vi "UI.vi"() -> ()   [LabVIEW 2017, in "TestLibrary.lvlib" / "GSharpCls.lvclass"]
uses:
  GSharpCls.lvclass
  Enum.ctl
panel:
  out "error out":errorcluster
  in  "Enum":T1
  out "Numeric out":dbl
  out "String":string
  in  "Numeric":dbl
  in  "stop":bool
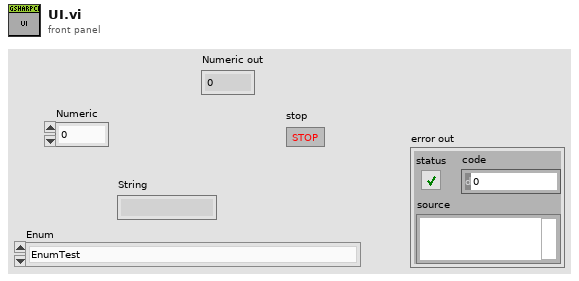
[diagram p1: front panel]
types:
  T1 = typedef "TestLibrary.lvlib/GSharpCls.lvclass/Enum.ctl" = enum16{"EnumTest", "EnumTest2"}
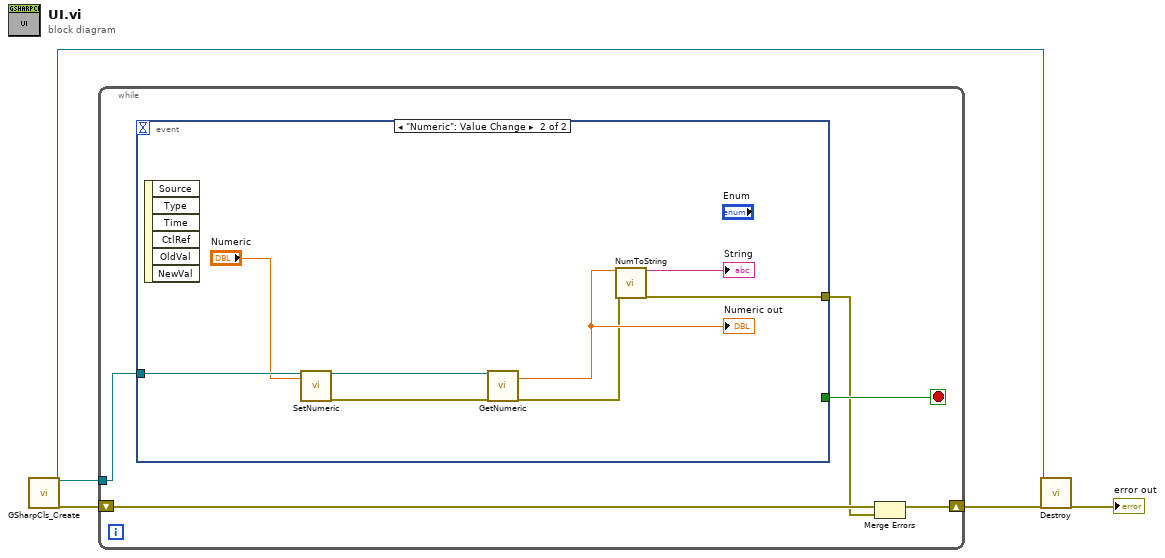
[diagram p0: block diagram]
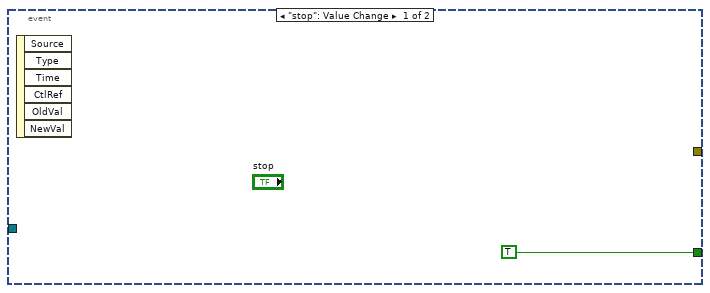
[diagram p2: hidden frame]
diagram:
  n1 = call "GSharpCls_Create.vi"() -> ("reference out"=w3:refnum<class "GSharpCls.lvclass">, "error out"=w4:errorcluster)  [unwired: 18 in]
  n2 = while {
    tunnel: w3 -> [w5]
    shift-right: [w7] -> w2
    shift-left: w4 -> [w8]
    stop <- w9 stop-if-true
    n3 = event shown="[1] \"Numeric\": Value Change" {
      selector: _ -> [_ _]
      dyn-events: _ -> [_ _]
      timeout: _ -> [_ _]
      tunnel: [TRUE _] -> w9
      tunnel: [_ w17] -> w6
      tunnel: w5 -> [_ w16]
      event "stop": Value Change {
        n4 = event-data() -> ()  [unwired: 1 in, 6 out]
      }
      event "Numeric": Value Change {
        n5 = event-data() -> ()  [unwired: 1 in, 6 out]
        n6 = call-dynamic "SetNumeric.vi"("reference in"=w16, "Numeric"="Numeric") -> ("reference out"=w11:refnum<class "GSharpCls.lvclass">, "error out"=w13:errorcluster)  [unwired: 16 in]
        n7 = call-dynamic "GetNumeric.vi"("reference in"=w11, "error in (no error)"=w13) -> ("Numeric"=w14:dbl, "error out"=w12:errorcluster)  [unwired: 15 in, 1 out]
        "Numeric out" <- w14
        n8 = call "NumToString.vi"("Numeric"=w14, "error in (no error)"=w12) -> ("String"=→"String":string, "error out"=w17:errorcluster)  [unwired: 16 in]
      }
    }
    n9 = Merge Errors(w8, w6) -> (w7:errorcluster)
  }
  n10 = call-dynamic "Destroy.vi"("reference in"=w3, "error in (no error)"=w2) -> ("error out"=→"error out":errorcluster)  [unwired: 16 in, 1 out]
